vi "PSK_Mod_Receive_test.vi"() -> ()   [LabVIEW 2014]
uses:
  <vilib>/addons/Modulation/Digital/General/MT Generate Bits (Galois, PN Order).vi
  <vilib>/addons/Modulation/Digital/Support/Common/Validators/mod_Generate Bits Validate.vi
  <vilib>/addons/Modulation/Analog/support/mod_Set Error Source.vi
  <vilib>/addons/Modulation/Digital/General/MT Generate PSK System Parameters(M).vi
  <vilib>/addons/Modulation/Digital/Support/Common/Validators/mod_Generate Filter Coefficients Validate.vi
  <vilib>/addons/Modulation/Digital/General/subVIs/mod_Generate Filter Coefficients.vi
  <vilib>/addons/Modulation/Digital/General/subVIs/mod_Generate Bits PN Sequence.vi
  <vilib>/addons/Modulation/Digital/General/MT Generate PSK Synchronization Parameters (bit array).vi
  <instrlib>/niUSRP/niUSRP Fetch Rx Data (CDB Cluster).vi
  <vilib>/addons/Modulation/niDMT.lvlib
  <vilib>/addons/Modulation/niAMT.lvlib
panel:
  in  "output bit stream 3":i8[](array[numeric]) caption="output bit stream"
  out "Packets received":i32
  out "bits received":i32
  out "Rx Symbol time":dbl
  out "Array":i8[][](array[numeric])
  in  "Message bits":i32=128
  in  "Sync bits":i32=20
  out "sync correct?":bool
  out "output bit stream":i8[](array[numeric])
  out "Before demod&compensation":waveform(dbl)(graph)
  in  "stop":bool
  out "Constellation Graph":T1(graph) caption="Tx Signal Constellation"
  out "error out":errorcluster={"status"=FALSE, "code"=1074118647, "source"="niUSRP Fetch Rx Data (CDB Cluster).vi<ERR>Overflow: an internal receive buffer has filled before the data could be returned.  Consider reducing the IQ rate, increasing the Fetch rate, or increasing the number of samples per Fetch."}
  in  "USRP IP Address":refnum<k15>="192.168.10.1"
  out "Actual Rx Parameters":T2={"Rx IQ Sampling\nRate [s/sec]"=200000.0, "Rx\nFrequency [Hz]"=915000000.0, "Rx Gain [dB]"=20.0, "Rx Antenna"="RX1"} {"Rx Gain [dB]" format="%#.6p"; "Rx\nFrequency [Hz]" format="%#.6p"; "Rx IQ Sampling\nRate [s/sec]" format="%#.6p"}
  in  "Rx Parameters":T2={"Rx IQ Sampling\nRate [s/sec]"=400000.0, "Rx\nFrequency [Hz]"=5795000000.0, "Rx Gain [dB]"=0.0, "Rx Antenna"="RX1"} {"Rx Gain [dB]" format="%#.6p"; "Rx\nFrequency [Hz]" format="%#.6p"; "Rx IQ Sampling\nRate [s/sec]" format="%#.6p"}
  in  "Acquisition Duration [sec]":dbl=0.04 format="%#.6p"
  in  "Guard bits":i32=20
  in  "filter parameters":T3={"Alpha"=0.5, "Filter Length"=6, "TX Filter"=enum."Root Raised Cos"} {"Alpha" format="%.2f"}
  in  "QPSK System Parameters":T4={"Samples per Symbol"=8, "symbol map"=[], "Differential PSK"=enum."disable", "PSK type"=0} {"PSK type" items=["normal", "shifted", "offset"]; "symbol map" format="%.3f"}
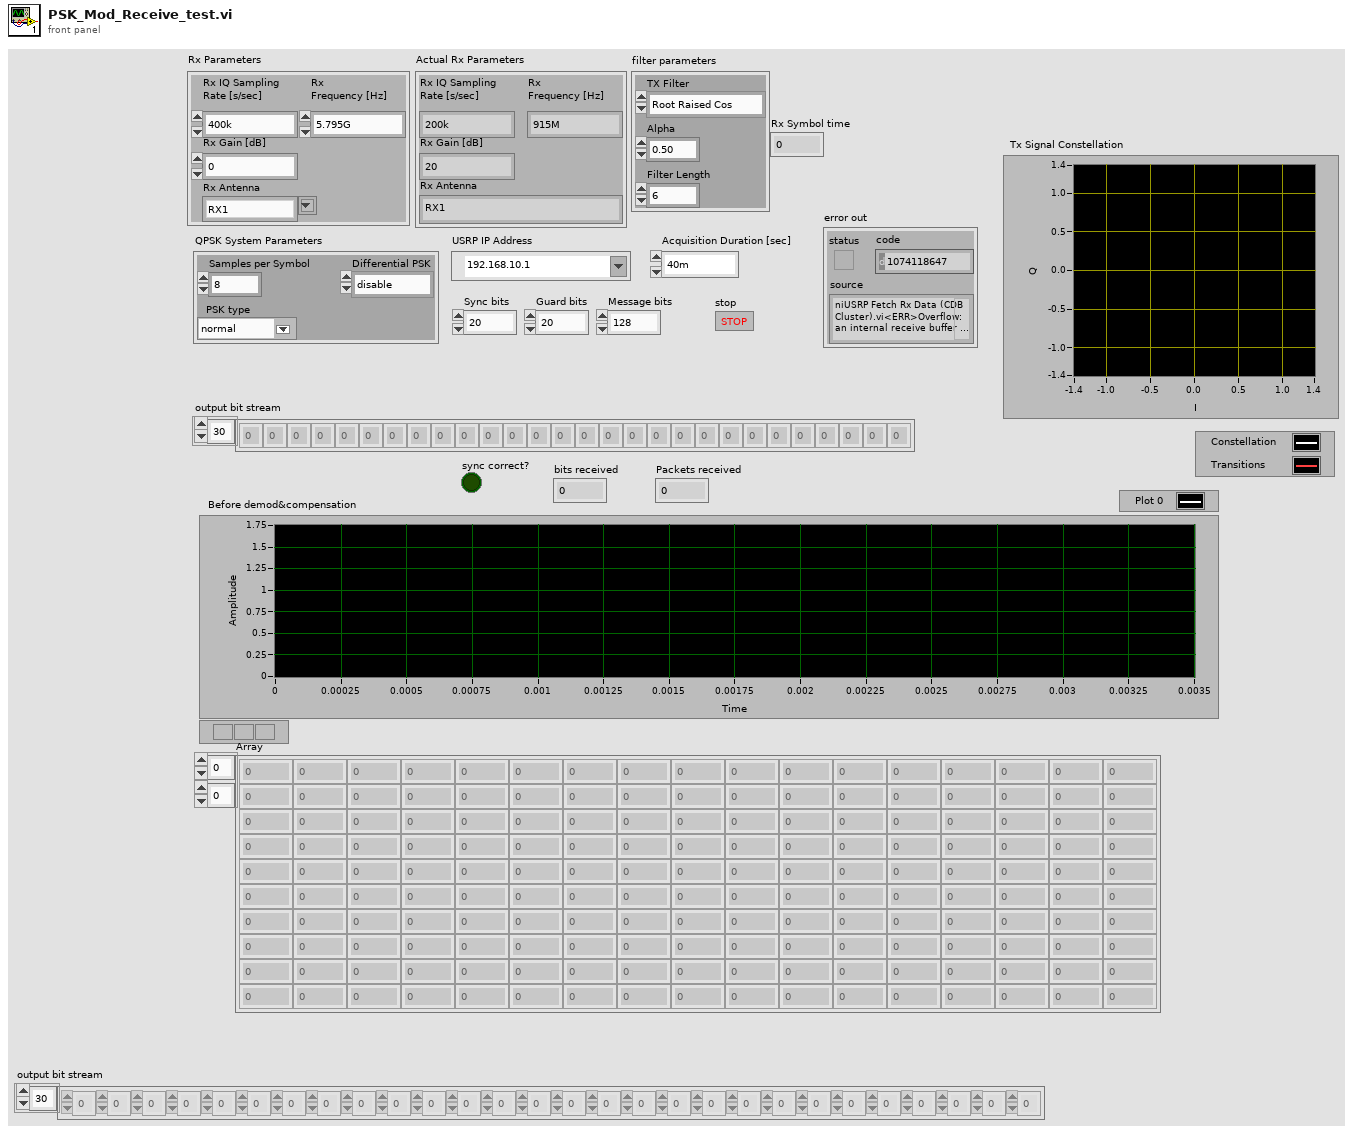
[diagram p1: front panel]
types:
  T1 = cluster{"constellation":dbl[], "oversampled data":dbl[]}[]
  T2 = cluster{"Rx IQ Sampling\nRate [s/sec]":dbl, "Rx\nFrequency [Hz]":dbl, "Rx Gain [dB]":dbl, "Rx Antenna":string}
  T3 = cluster{"Alpha":dbl, "Filter Length":i32, "TX Filter":enum16{"none", "Raised Cosine", "Root Raised Cos", "Gaussian"}}
  T4 = cluster{"Samples per Symbol":i32, "symbol map":cdb[], "Differential PSK":enum16{"disable", "enable"}, "PSK type":u16}
  T5 = enum16{"FSK", "PSK", "QAM", "MSK", "PAM", "ASK", "CPM"}
  T6 = enum16{"none", "Raised Cosine", "Root Raised Cos", "Gaussian"}
  T7 = cluster{"samples per symbol (16)":i32, "symbol map":cdb[], "differential PSK":enum16{"disable", "enable"}, "PSK type":u16}
  T8 = cluster{"expected sync location (symbols)":i32, "sync sequence":cdb[], "sync location uncertainty (symbols)":i32, "sync indent (symbols)":i32}
  T9 = typedef "niAMT.lvlib/Complex Data Waveform.ctl" = cluster{"t0":dbl, "dt":dbl, "Y":cdb[]}
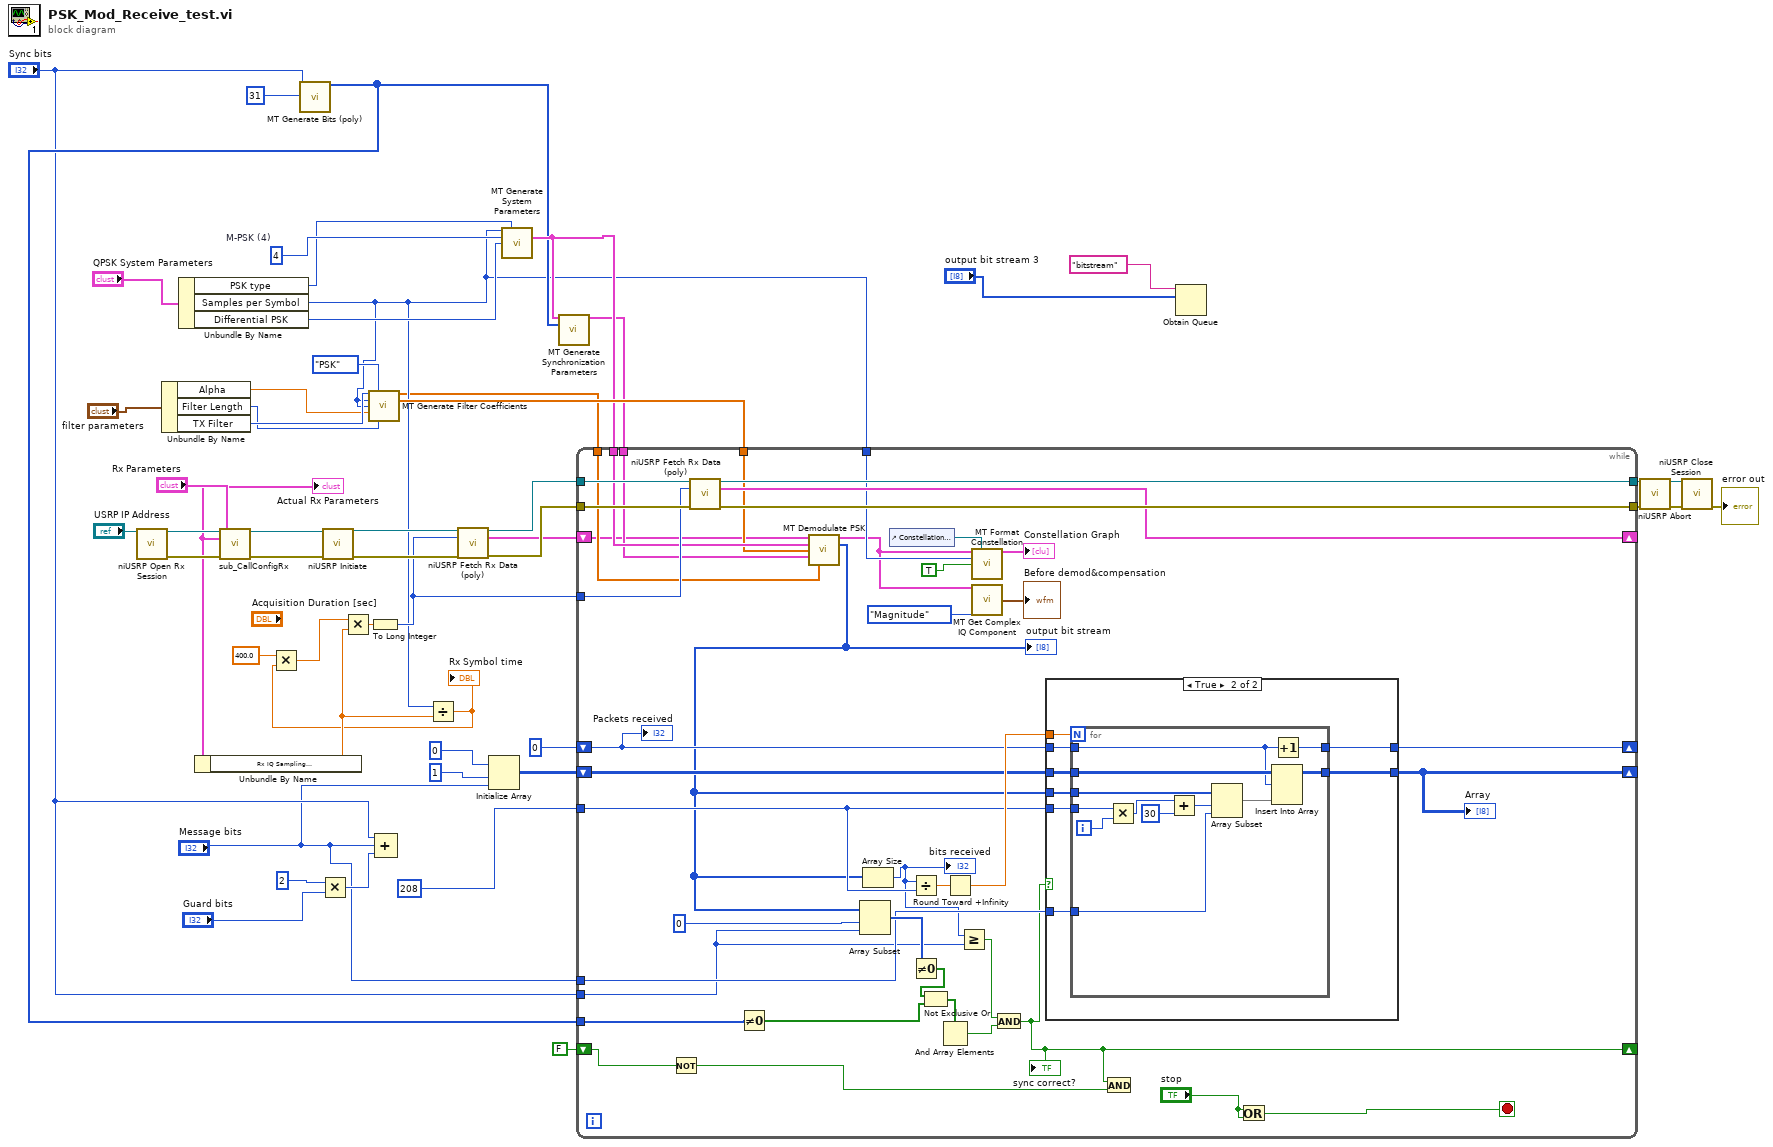
[diagram p0: block diagram]
diagram:
  w50 = 4  # M-PSK (4)
  n1 = call <instrlib>:"niUSRP Open Rx Session.vi"("device names"="USRP IP Address") -> ("session handle out"=w41:refnum<k15>, "error out"=w42:errorcluster)  [unwired: 13 in]
  n2 = Unbundle By Name("filter parameters") -> ("Alpha"=w47:dbl, "Filter Length"=w48:i32, "TX Filter"=w49:T6)
  n3 = Unbundle By Name("QPSK System Parameters") -> ("PSK type"=w23:u16, "Samples per Symbol"=w14:i32, "Differential PSK"=w51:enum16{"disable", "enable"})
  n4 = call "sub_CallConfigRx.vi"("session handle"=w41, "Rx Parameters"="Rx Parameters", "error in"=w42) -> ("session handle out"=w39:refnum<k15>, "Actual Rx Parameters"=w36:T2, "error out"=w38:errorcluster)  [unwired: 10 in]
  "Actual Rx Parameters" <- w36
  n5 = Unbundle By Name(w36) -> ("Rx IQ Sampling\nRate [s/sec]"=w13:dbl)
  n6 = call-poly <vilib>:"MT Generate Bits (poly).vi"("total bits (128)"="Sync bits", "PN sequence order (9)"=31) -> ("output bit stream"=w20:i8[])  [unwired: 11 in, 2 out]
  n7 = Multiply(x=2, y="Guard bits") -> (x*y=w16:i32)
  n8 = call <instrlib>:"niUSRP Initiate.vi"("session handle"=w39, "error in (no error)"=w38) -> ("session handle out"=w35:refnum<k15>, "error out"=w34:errorcluster)  [unwired: 12 in]
  n9 = call <vilib>:"MT Generate Filter Coefficients.vi"("pulse shaping filter (none)"=w49, "modulation type"=T5."PSK", "pulse shaping samples per symbol (16)"=w14, "matched samples per symbol (16)"=w14, "filter parameter"=w47, "filter length (symbols)"=w48) -> ("pulse shaping filter coefficients"=w8:dbl[], "matched filter coefficients"=w24:dbl[])  [unwired: 7 in, 1 out]
  n10 = Compound Arithmetic op=ADD("Sync bits", "Message bits", w16) -> ()  [unwired: 1 out]
  n11 = Divide(x=w14, y=w13) -> (x/y=w11:dbl)
  "Rx Symbol time" <- w11
  n12 = Multiply(x=400.0, y=w11) -> (x*y=w10:dbl)
  n13 = Multiply(x=w10, y=w13) -> (x*y=w43:dbl)
  n14 = To Long Integer(number=w43) -> (32bit integer=w26:i32)
  n15 = call-poly <instrlib>:"niUSRP Fetch Rx Data (poly).vi"("session handle"=w35, "number of samples"=w26, "error in (no error)"=w34) -> ("session handle out"=w30:refnum<k15>, "data"=w25:cluster{"t0":dbl, "dt":dbl, "Y":cdb[]}, "error out"=w27:errorcluster)  [unwired: 9 in, 1 out]
  n16 = Initialize Array(i8 0 ("element"), 1 ("dimension size"), "Message bits") -> (w5:i8[][])
  n17 = call-poly <vilib>:"MT Generate System Parameters.vi"("samples per symbol (16)"=w14, "PSK type"=w23, "M-PSK (4)"=w50, "differential PSK"=w51) -> ("PSK system parameters"=w22:T7)  [unwired: 9 in, 2 out]
  n18 = call-poly <vilib>:"MT Generate Synchronization Parameters.vi"("PSK system parameters"=w22, "sync bits"=w20) -> ("PSK synchronization parameters"=w21:T8)  [unwired: 12 in, 1 out]
  n19 = while {
    tunnel: w30 -> [w94]
    tunnel: [w93] -> w29
    tunnel: [w92] -> w28
    tunnel: w27 -> [w91]
    tunnel: w26 -> [w90]
    shift-right: [w89] -> _
    shift-left: w25 -> [w53]
    tunnel: w14 -> [w86]
    tunnel: w24 -> [w83]
    tunnel: w22 -> [w84]
    tunnel: w21 -> [w82]
    tunnel: "Sync bits" -> [w64]
    tunnel: w20 -> [w79]
    tunnel: 208 -> [w71]
    tunnel: "Message bits" -> [w69]
    shift-right: [w60] -> _
    shift-left: FALSE -> [w68]
    tunnel: w8 -> [w61]
    shift-right: [w58] -> _
    shift-left: 0 -> [w59]
    shift-right: [w55] -> _
    shift-left: w5 -> [w56]
    stop <- w66 stop-if-true
    n20 = Not(x=w68) -> (.not. x?=w67:bool)
    n21 = call-poly <instrlib>:"niUSRP Fetch Rx Data (poly).vi"("session handle"=w94, "number of samples"=w90, "error in (no error)"=w91) -> ("session handle out"=w93:refnum<k15>, "data"=w89:cluster{"t0":dbl, "dt":dbl, "Y":cdb[]}, "error out"=w92:errorcluster)  [unwired: 9 in, 1 out]
    n22 = Not Equal To 0?(x=w79) -> (x != 0?=w76:bool[])
    n23 = call <vilib>:"MT Demodulate PSK.vi"("input complex waveform"=w53, "PSK system parameters"=w84, "matched filter coefficients"=w83, "synchronization parameters"=w82, "pulse shaping filter coefficients"=w61) -> ("recovered complex waveform"=w74:T9, "output bit stream"=w54:i8[])  [unwired: 6 in, 3 out]
    "output bit stream" <- w54
    n24 = Array Subset(array=w54, index=0, length=w64) -> (w80:i8[])
    n25 = Array Size(array=w54) -> (size(s)=w65:i32)
    "bits received" <- w65
    n26 = control-ref of="Constellation Graph"() -> (w88:refnum<vi>)
    n27 = Divide(x=w65, y=w71) -> (x/y=w73:dbl)
    n28 = Not Equal To 0?(x=w80) -> (x != 0?=w77:bool[])
    n29 = Not Exclusive Or(1:w76, 2:w77) -> (0:w78:bool[])
    n30 = And Array Elements(Boolean array=w78) -> (logical AND=w62:bool)
    n31 = Round Toward +Infinity(x=w73) -> (ceil(x): smallest int >= x=w72:dbl)
    n32 = Greater Or Equal?(x=w65, y=w64) -> (x >= y?=w63:bool)
    n33 = call <vilib>:"MT Format Constellation.vi"("waveform"=w74, "constellation reference"=w88, "samples per symbol"=w86, "autoscale"=TRUE) -> ("constellation graph"=→"Constellation Graph":T1)  [unwired: 10 in, 1 out]
    n34 = call <vilib>:"MT Get Complex IQ Component.vi"("IQ data (complex) in"=w74, "component choice"=enum16{"I", "Q", "Magnitude", "Phase"}."Magnitude") -> ("CE component"=→"Before demod&compensation":waveform(dbl))  [unwired: 11 in, 2 out]
    n35 = And(x=w63, y=w62) -> (x .and. y?=w60:bool)
    "sync correct?" <- w60
    n36 = case shown="True" w60 {
      tunnel: w72 -> [_ w104]
      tunnel: w54 -> [_ w103]
      tunnel: w71 -> [_ w102]
      tunnel: w69 -> [_ w101]
      tunnel: w59 -> [w96 w100]
      tunnel: [w96 w99] -> w58
      tunnel: [w95 w97] -> w55
      tunnel: w56 -> [w95 w98]
      frame False {
      }
      frame True {
        n37 = for {
          N: w104 -> [_]
          tunnel: w103 -> [w116]
          tunnel: w102 -> [w114]
          tunnel: w101 -> [w113]
          tunnel: w100 -> [w105]
          tunnel: [w106] -> w99
          tunnel: w98 -> [w109]
          tunnel: [w108] -> w97
          i -> [w115]
          n38 = Multiply(x=w114, y=w115) -> (x*y=w112:i32)
          n39 = Add(x=w112, y=30) -> (x+y=w110:i32)
          n40 = Array Subset(array=w116, index=w110, length=w113) -> (w107:i8[])
          n41 = Insert Into Array(array=w109, index (row)=w105, new element=w107) -> (w108:i8[][])  [unwired: 1 in]
          n42 = Increment(x=w105) -> (x+1=w106:i32)
        }
      }
    }
    "Array" <- w55
    n43 = And(x=w60, y=w67) -> ()  [unwired: 1 out]
    n44 = Or(x="stop", y="stop") -> (x .or. y?=w66:bool)
    "Packets received" <- w59
  }
  n45 = Obtain Queue(name (unnamed)="bitstream", element data type="output bit stream 3") -> ()  [unwired: 3 in, 3 out]
  n46 = call <instrlib>:"niUSRP Abort.vi"("session handle"=w29, "error in (no error)"=w28) -> ("session handle out"=w32:refnum<k15>, "error out"=w33:errorcluster)  [unwired: 12 in]
  n47 = call <instrlib>:"niUSRP Close Session.vi"("session handle"=w32, "error in (no error)"=w33) -> ("error out"=→"error out":errorcluster)  [unwired: 13 in]
